vi "Emballage nom fichier utilisable.vi"(1 "chaîne en entrée":string) -> (0 "chaîne résultante":string)   [LabVIEW 2020]
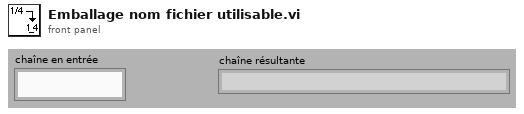
[diagram p1: front panel]
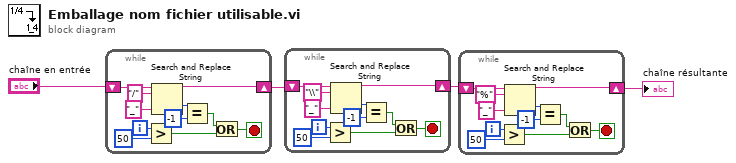
[diagram p0: block diagram]
diagram:
  n1 = while {
    shift-right: [w11] -> w3
    shift-left: "chaîne en entrée" -> [w12]
    i -> [w9]
    stop <- w5 stop-if-true
    n2 = Greater?(x=w9, y=50) -> (0:w7:bool)
    n3 = Search and Replace String(input string=w12, search string="/" ("chaîne recherchée"), replace string="_" ("chaîne de remplacement (\"\")")) -> (result string=w11:string, offset past replacement=w14:i32)  [unwired: 5 in, 2 out]
    n4 = Equal?(x=w14, y=-1) -> (x = y?=w6:bool)
    n5 = Or(x=w6, y=w7) -> (x .or. y?=w5:bool)
  }
  n6 = while {
    shift-right: [w22] -> w1
    shift-left: w3 -> [w23]
    i -> [w20]
    stop <- w16 stop-if-true
    n7 = Greater?(x=w20, y=50) -> (0:w18:bool)
    n8 = Search and Replace String(input string=w23, search string="\\" ("chaîne recherchée"), replace string="_" ("chaîne de remplacement (\"\")")) -> (result string=w22:string, offset past replacement=w25:i32)  [unwired: 5 in, 2 out]
    n9 = Equal?(x=w25, y=-1) -> (x = y?=w17:bool)
    n10 = Or(x=w17, y=w18) -> (x .or. y?=w16:bool)
  }
  n11 = while {
    shift-right: [w33] -> w2
    shift-left: w1 -> [w34]
    i -> [w31]
    stop <- w27 stop-if-true
    n12 = Greater?(x=w31, y=50) -> (0:w29:bool)
    n13 = Search and Replace String(input string=w34, search string="%" ("chaîne recherchée"), replace string="_" ("chaîne de remplacement (\"\")")) -> (result string=w33:string, offset past replacement=w36:i32)  [unwired: 5 in, 2 out]
    n14 = Equal?(x=w36, y=-1) -> (x = y?=w28:bool)
    n15 = Or(x=w28, y=w29) -> (x .or. y?=w27:bool)
  }
  "chaîne résultante" <- w2
